vi "init.vi"(8 "error in (no error)":errorcluster, 11 "PressureValve in":refnum<class "PressureValve.lvclass">) -> (0 "error out":errorcluster, 3 "PressureValve out":refnum<class "PressureValve.lvclass">)   [LabVIEW 2015, in "PressureValve.lvlib" / "PressureValve.lvclass"]
uses:
  <userlib>/Common/Devices/PressureValve/PressureValve/PressureValve.lvclass
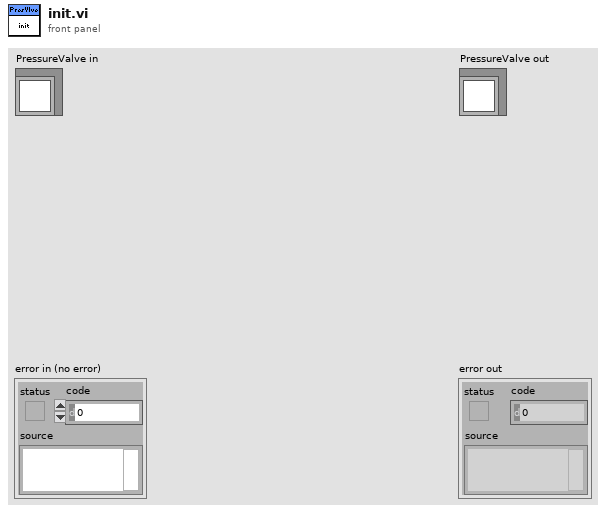
[diagram p1: front panel]
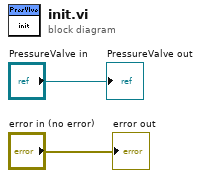
[diagram p0: block diagram]
diagram:
  "error out" <- "error in (no error)"
  "PressureValve out" <- "PressureValve in"
